vi "Main.vi"() -> ()   [LabVIEW 2019]
uses:
  Controls/Enum/Supervisor_Enum.ctl
  Controls/Enum/DAQ_Enum.ctl
  Controls/Clust/DAQ Clust.ctl
panel:
  in  "Exit":bool
  in  "stop":bool
  in  "Start":bool
  out "System Time":string
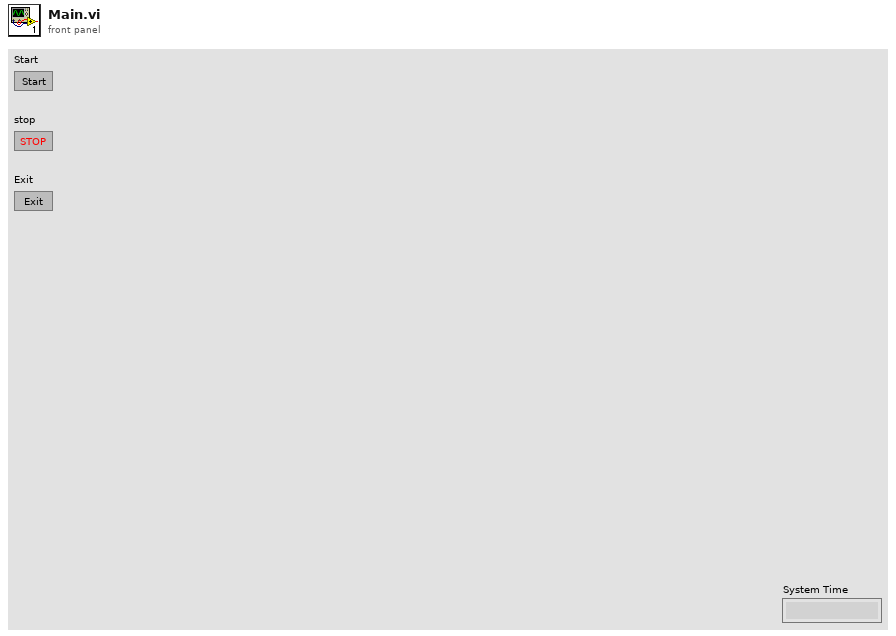
[diagram p1: front panel]
types:
  T1 = typedef "DAQ Clust.ctl" = cluster{"Acquisition Task":refnum<k21>}
  T2 = typedef "DAQ_Enum.ctl" = enum16{"DAQ_Init", "DAQ_Start", "DAQ_Read", "DAQ_Stop", "DAQ_Close"}
  T3 = typedef "Supervisor_Enum.ctl" = enum16{"Spvsr_Init", "Spvsr_Start", "Spvsr_Stop", "Spvsr_Close"}
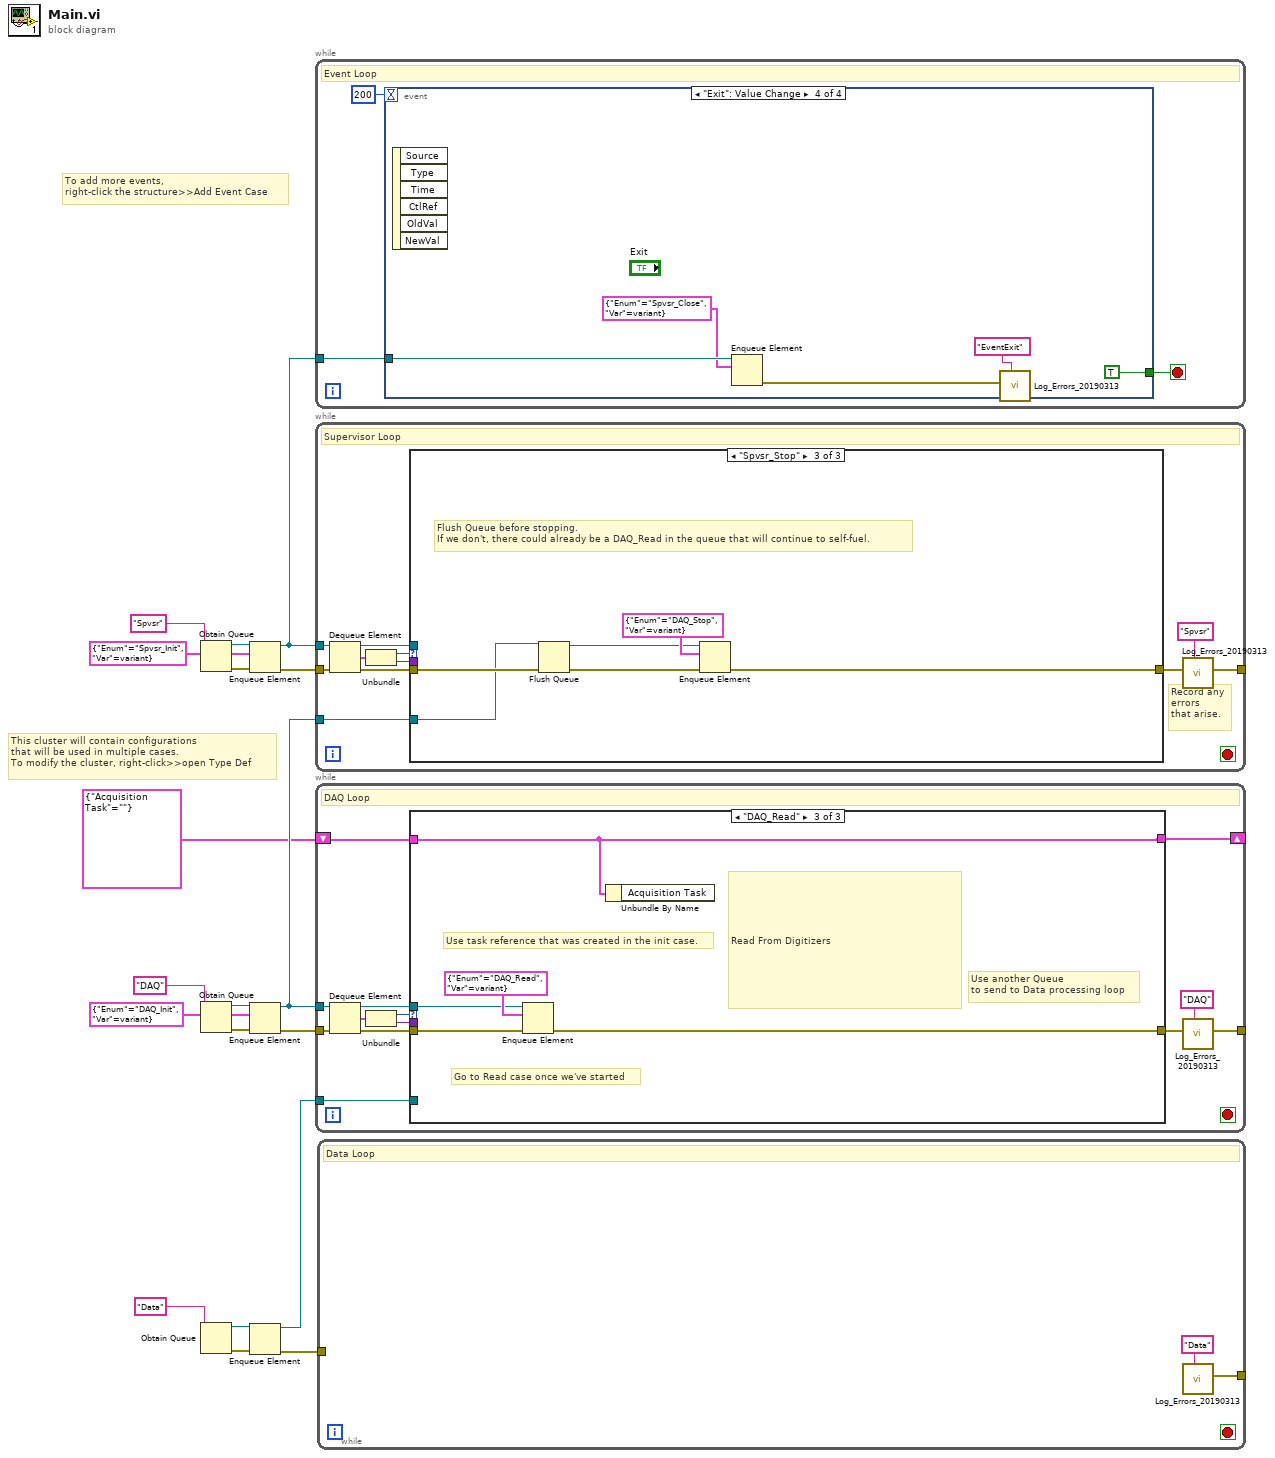
[diagram p0: block diagram]
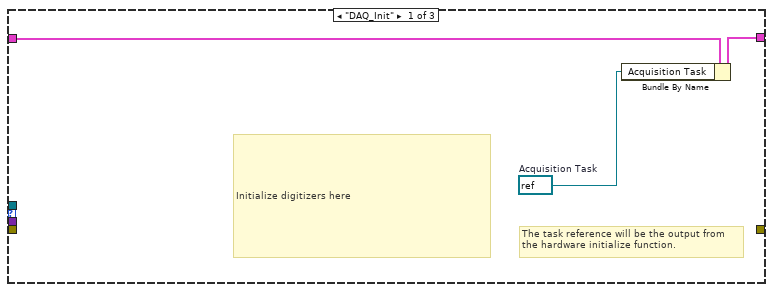
[diagram p2: hidden frame]
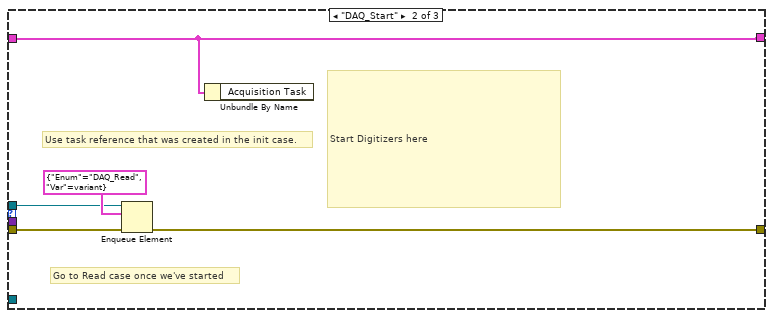
[diagram p3: hidden frame]
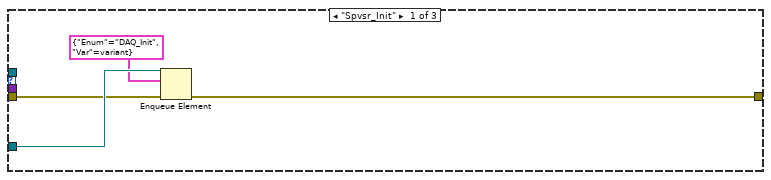
[diagram p4: hidden frame]
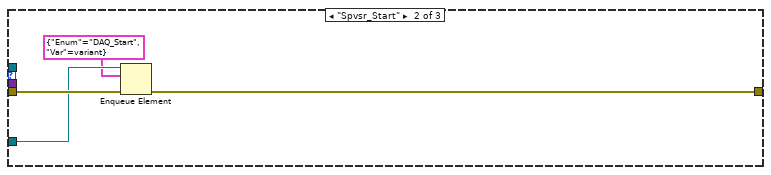
[diagram p5: hidden frame]
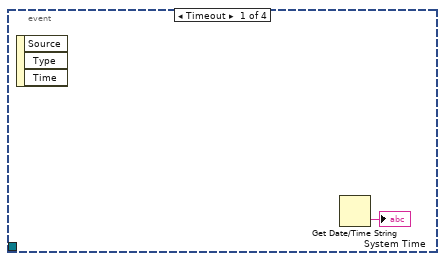
[diagram p6: hidden frame]
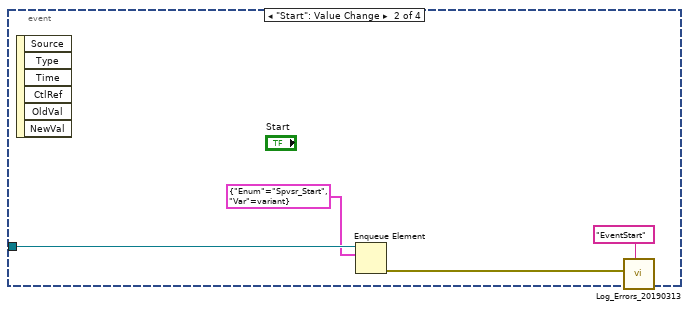
[diagram p7: hidden frame]
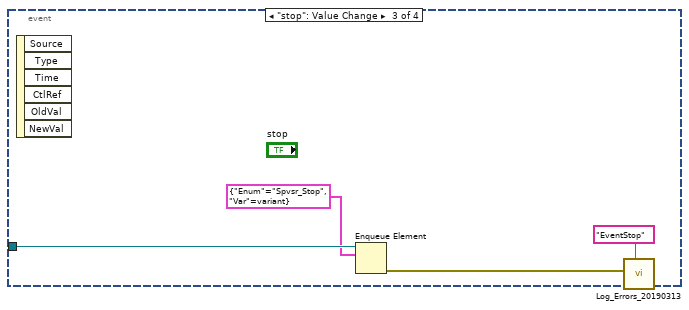
[diagram p8: hidden frame]
diagram:
  w14 = cluster{"Enum":T2, "Var":variant} {"Enum"=enum."DAQ_Init", "Var"=variant}
  w16 = cluster{"Enum":T3, "Var":variant} {"Enum"=enum."Spvsr_Init", "Var"=variant}
  # "To add more events,\nright-click the structure>>Add Event Case"
  # "This cluster will contain configurations\nthat will be used in multiple cases.\nTo modify the cluster, right-click>>open Type Def"
  n1 = Obtain Queue(name (unnamed)="Spvsr", element data type=w16) -> (queue out=w17:refnum<queue>, error out=w19:errorcluster)  [unwired: 3 in, 1 out]
  n2 = Obtain Queue(name (unnamed)="DAQ", element data type=w14) -> (queue out=w13:refnum<queue>, error out=w11:errorcluster)  [unwired: 3 in, 1 out]
  n3 = Obtain Queue(name (unnamed)="Data") -> (queue out=w7:refnum<queue>, error out=w8:errorcluster)  [unwired: 4 in, 1 out]
  n4 = Enqueue Element(queue=w17, element=w16, error in (no error)=w19) -> (queue out=w15:refnum<queue>, error out=w18:errorcluster)  [unwired: 1 in, 1 out]
  n5 = Enqueue Element(queue=w13, element=w14, error in (no error)=w11) -> (queue out=w10:refnum<queue>, error out=w12:errorcluster)  [unwired: 1 in, 1 out]
  n6 = Enqueue Element(queue=w7, error in (no error)=w8) -> (element=w6:cluster{"Enum":T2, "Var":variant}, queue out=w4:refnum<queue>, error out=w5:errorcluster)  [unwired: 1 in, 1 out]
  n7 = while {
    tunnel: w15 -> [w21]
    stop <- w20 stop-if-true
    # "Event Loop"
    n8 = event shown="[3] \"Exit\": Value Change" {
      selector: _ -> [_ _ _ _]
      dyn-events: _ -> [_ _ _ _]
      timeout: 200 -> [_ _ _ _]
      tunnel: w21 -> [_ w27 w31 w36]
      tunnel: [_ _ _ TRUE] -> w20
      event Timeout {
        n9 = event-data() -> ()  [unwired: 1 in, 3 out]
        n10 = Get Date/Time String() -> (time string=→"System Time":string)  [unwired: 3 in, 1 out]
      }
      event "Start": Value Change {
        n11 = event-data() -> ()  [unwired: 1 in, 6 out]
        n12 = Enqueue Element(queue=w27, element=cluster{"Enum":T3, "Var":variant} {"Enum"=enum."Spvsr_Start", "Var"=variant}) -> (error out=w24:errorcluster)  [unwired: 2 in, 2 out]
        n13 = call "Log_Errors_20190313.vi"("LoopName"="EventStart", "error in"=w24) -> ()  [unwired: 9 in, 1 out]
      }
      event "stop": Value Change {
        n14 = event-data() -> ()  [unwired: 1 in, 6 out]
        n15 = Enqueue Element(queue=w31, element=cluster{"Enum":T3, "Var":variant} {"Enum"=enum."Spvsr_Stop", "Var"=variant}) -> (error out=w28:errorcluster)  [unwired: 2 in, 2 out]
        n16 = call "Log_Errors_20190313.vi"("LoopName"="EventStop", "error in"=w28) -> ()  [unwired: 9 in, 1 out]
      }
      event "Exit": Value Change {
        n17 = event-data() -> ()  [unwired: 1 in, 6 out]
        n18 = Enqueue Element(queue=w36, element=cluster{"Enum":T3, "Var":variant} {"Enum"=enum."Spvsr_Close", "Var"=variant}) -> (error out=w33:errorcluster)  [unwired: 2 in, 2 out]
        n19 = call "Log_Errors_20190313.vi"("LoopName"="EventExit", "error in"=w33) -> ()  [unwired: 9 in, 1 out]
      }
    }
  }
  n20 = while {
    tunnel: w18 -> [w47]
    tunnel: w15 -> [w45]
    tunnel: w10 -> [w40]
    tunnel: [w37] -> _
    stop <- _ stop-if-true
    # "Record any\nerrors \nthat arise."
    # "Supervisor Loop"
    n21 = Dequeue Element(queue=w45, error in (no error)=w47) -> (queue out=w43:refnum<queue>, element=w44:cluster{"Enum":T3, "Var":variant}, error out=w46:errorcluster)  [unwired: 1 in, 1 out]
    n22 = Unbundle(w44) -> ("Enum"=w42:T3, "Var"=w41:variant)
    n23 = case shown="\"Spvsr_Stop\"" w42 {
      tunnel: w46 -> [w50 w55 w58]
      tunnel: w43 -> [_ _ _]
      tunnel: w41 -> [_ _ _]
      tunnel: w40 -> [w51 w53 w56]
      tunnel: [w48 w54 w61] -> w38
      frame "Spvsr_Init" {
        n24 = Enqueue Element(queue=w51, element=cluster{"Enum":T2, "Var":variant} {"Enum"=enum."DAQ_Init", "Var"=variant}, error in (no error)=w50) -> (error out=w48:errorcluster)  [unwired: 1 in, 2 out]
      }
      frame "Spvsr_Start" {
        n25 = Enqueue Element(queue=w53, element=cluster{"Enum":T2, "Var":variant} {"Enum"=enum."DAQ_Start", "Var"=variant}, error in (no error)=w55) -> (error out=w54:errorcluster)  [unwired: 1 in, 2 out]
      }
      frame "Spvsr_Stop" {
        # "Flush Queue before stopping.\nIf we don't, there could already be a DAQ_Read in the queue that will continue to self-fuel."
        n26 = Flush Queue(queue=w56, error in (no error)=w58) -> (queue out=w57:refnum<queue>, error out=w59:errorcluster)  [unwired: 1 out]
        n27 = Enqueue Element(queue=w57, element=cluster{"Enum":T2, "Var":variant} {"Enum"=enum."DAQ_Stop", "Var"=variant}, error in (no error)=w59) -> (error out=w61:errorcluster)  [unwired: 1 in, 2 out]
      }
    }
    n28 = call "Log_Errors_20190313.vi"("LoopName"="Spvsr", "error in"=w38) -> ("error out"=w37:errorcluster)  [unwired: 9 in]
  }
  n29 = while {
    tunnel: w12 -> [w74]
    tunnel: w10 -> [w72]
    shift-right: [w65] -> _
    shift-left: T1 {"Acquisition Task"=""} ("DAQ Clust") -> [w66]
    tunnel: [w63] -> _
    tunnel: w4 -> [w62]
    stop <- _ stop-if-true
    # "DAQ Loop"
    n30 = Dequeue Element(queue=w72, error in (no error)=w74) -> (queue out=w70:refnum<queue>, element=w71:cluster{"Enum":T2, "Var":variant}, error out=w73:errorcluster)  [unwired: 1 in, 1 out]
    n31 = Unbundle(w71) -> ("Enum"=w69:T2, "Var"=w68:variant)
    n32 = case shown="\"DAQ_Read\"" w69 {
      tunnel: w73 -> [_ w79 w85]
      tunnel: w70 -> [_ w80 w86]
      tunnel: w68 -> [_ _ _]
      tunnel: w66 -> [w77 w82 w88]
      tunnel: [w76 w82 w88] -> w65
      tunnel: [_ w78 w84] -> w64
      tunnel: w62 -> [_ _ w83]
      frame "DAQ_Init" {
        w75 = refnum<k21> refnum  # Acquisition Task
        # "The task reference will be the output from\nthe hardware initialize function."
        # "Initialize digitizers here"
        n33 = Bundle By Name(cluster=w77, "Acquisition Task"=w75) -> (w76:T1)
      }
      frame "DAQ_Start" {
        # "Go to Read case once we've started"
        # "Use task reference that was created in the init case."
        # "Start Digitizers here"
        n34 = Enqueue Element(queue=w80, element=cluster{"Enum":T2, "Var":variant} {"Enum"=enum."DAQ_Read", "Var"=variant}, error in (no error)=w79) -> (error out=w78:errorcluster)  [unwired: 1 in, 2 out]
        n35 = Unbundle By Name(w82) -> ()  [unwired: 1 out]
      }
      frame "DAQ_Read" {
        # "Use another Queue\nto send to Data processing loop"
        # "Go to Read case once we've started"
        # "Use task reference that was created in the init case."
        # "Read From Digitizers"
        n36 = Enqueue Element(queue=w86, element=cluster{"Enum":T2, "Var":variant} {"Enum"=enum."DAQ_Read", "Var"=variant}, error in (no error)=w85) -> (error out=w84:errorcluster)  [unwired: 1 in, 2 out]
        n37 = Unbundle By Name(w88) -> ()  [unwired: 1 out]
      }
    }
    n38 = call "Log_Errors_20190313.vi"("LoopName"="DAQ", "error in"=w64) -> ("error out"=w63:errorcluster)  [unwired: 9 in]
  }
  n39 = while {
    tunnel: w5 -> [_]
    tunnel: [w89] -> _
    stop <- _ stop-if-true
    # "Data Loop"
    n40 = call "Log_Errors_20190313.vi"("LoopName"="Data") -> ("error out"=w89:errorcluster)  [unwired: 10 in]
  }
